vi "WriteOrAppendToExcel.vi"(8 "Data":dbl[](array[numeric]), 9 "Column Headers":string[](array[string])=["Temperature"], 10 "Excel File Location":path, 11 "Excel Button":bool) -> ()   [LabVIEW 2020]
uses:
  <vilib>/Utility/file.llb/Write Delimited Spreadsheet (string).vi
  <vilib>/Utility/file.llb/Write Delimited Spreadsheet (DBL).vi
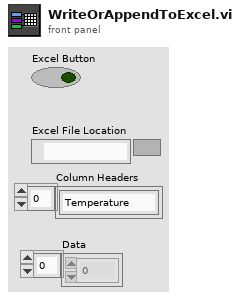
[diagram p1: front panel]
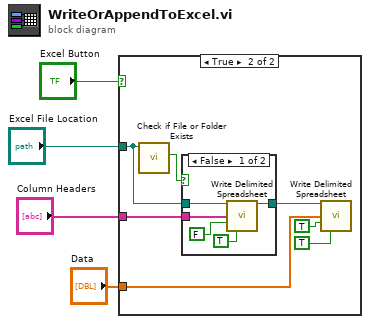
[diagram p0: block diagram]
diagram:
  n1 = case shown="True" "Excel Button" {
    tunnel: "Excel File Location" -> [_ w7]
    tunnel: "Data" -> [_ w6]
    tunnel: "Column Headers" -> [_ w5]
    frame False {
    }
    frame True {
      n2 = call <vilib>:"Check if File or Folder Exists.vi"("path"=w7) -> ("file or folder exists?"=w8:bool)  [unwired: 8 in, 2 out]
      n3 = case shown="False" w8 {
        tunnel: w7 -> [w16 w17]
        tunnel: [w14 w17] -> w11
        tunnel: w5 -> [w13 _]
        frame False {
          n4 = call-poly <vilib>:"Write Delimited Spreadsheet.vi"("file path (dialog if empty)"=w16, "1D data"=w13, "append to file? (new file:F)"=FALSE, "transpose? (no:F)"=TRUE) -> ("new file path (Not A Path if cancelled)"=w14:path)  [unwired: 10 in, 1 out]
        }
        frame True {
        }
      }
      n5 = call-poly <vilib>:"Write Delimited Spreadsheet.vi"("file path (dialog if empty)"=w11, "1D data"=w6, "append to file? (new file:F)"=TRUE, "transpose? (no:F)"=TRUE) -> ()  [unwired: 10 in, 2 out]
    }
  }
